vi "BandNoise Test Settings Get Configuration Data as String.vi"(8 "error in (no error)":errorcluster, 10 "Configuration Name":string, 11 "Band Noise Test Settings in":refnum<class "Band Noise Test Settings.lvclass">=refnum) -> (0 "error out":errorcluster, 1 "Reference Level":string, 2 "Frequency":string, 3 "Band Noise Test Settings out":refnum<class "Band Noise Test Settings.lvclass">, 4 "Span":string)   [LabVIEW 2016, in "Band Noise Test Settings.lvlib" / "Band Noise Test Settings.lvclass"]
uses:
  Band Noise Test Settings.lvclass
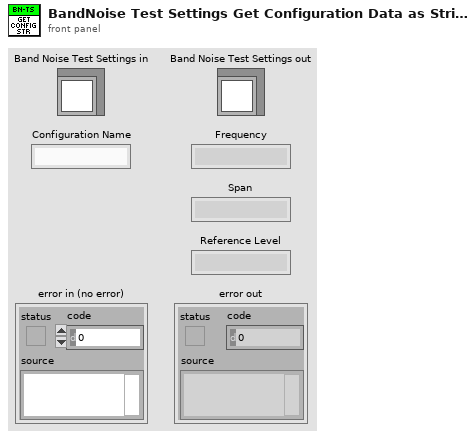
[diagram p1: front panel]
types:
  T1 = typedef "Band Noise Test Settings.lvlib/Band Noise Test Settings.lvclass/Band Noise Settings Cluster.ctl" = cluster{"Frequency":dbl, "Reference Level":dbl, "Span":dbl}
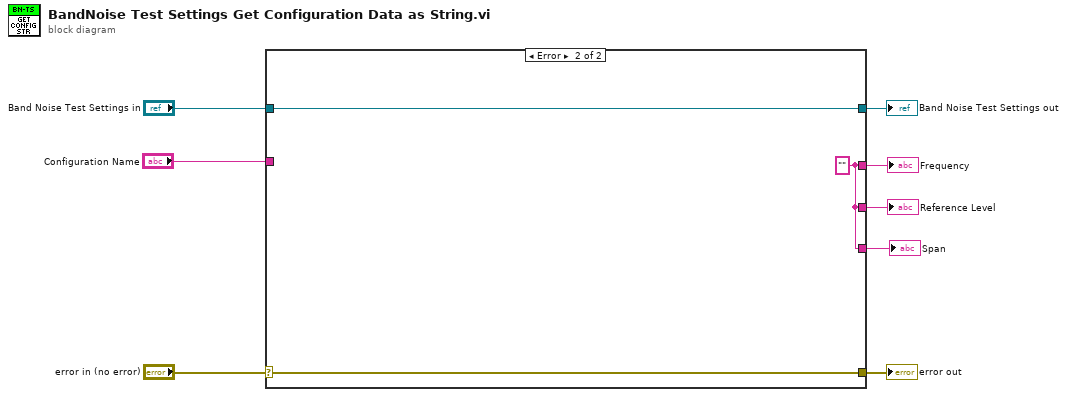
[diagram p0: block diagram]
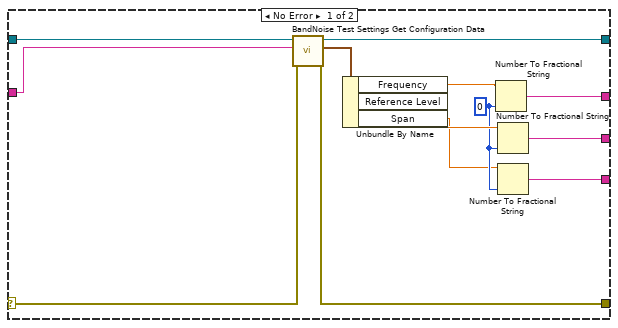
[diagram p2: hidden frame]
diagram:
  n1 = case shown="Error" "error in (no error)" {
    selector: "error in (no error)" -> [w18 w24]
    tunnel: [w21 w24] -> w7
    tunnel: [w19 w23] -> w5
    tunnel: "Band Noise Test Settings in" -> [w20 w23]
    tunnel: [w16 w22] -> w3
    tunnel: [w14 w22] -> w2
    tunnel: "Configuration Name" -> [w13 _]
    tunnel: [w9 w22] -> w1
    frame No Error {
      w11 = i16 0 ("precision (6)")
      n2 = call "BandNoise Test Settings Get Configuration Data.vi"("error in (no error)"=w18, "Configuration Name"=w13, "Band Noise Test Settings in"=w20) -> ("error out"=w21:errorcluster, "Band Noise Test Settings"=w12:T1, "Band Noise Test Settings out"=w19:refnum<class "Band Noise Test Settings.lvclass">)  [unwired: 6 in]
      n3 = Unbundle By Name(w12) -> ("Frequency"=w17:dbl, "Reference Level"=w15:dbl, "Span"=w10:dbl)
      n4 = Number To Fractional String(number=w17, precision (6)=w11) -> (F-format string=w16:string)  [unwired: 2 in]
      n5 = Number To Fractional String(number=w15, precision (6)=w11) -> (F-format string=w14:string)  [unwired: 2 in]
      n6 = Number To Fractional String(number=w10, precision (6)=w11) -> (F-format string=w9:string)  [unwired: 2 in]
    }
    frame Error {
      w22 = ""
    }
  }
  "error out" <- w7
  "Band Noise Test Settings out" <- w5
  "Frequency" <- w3
  "Reference Level" <- w2
  "Span" <- w1
